vi "LateralControl.vi"(6 "output range":cluster{"output high":dbl, "output low":dbl}, 7 "PID Gains lateral":T1={"proportional gain (Kc)"=0.008, "integral time (Ti, min)"=0.0, "derivative time (Td, min)"=-0.07}, 9 "Waypoint 0":dbl[](array[numeric]), 10 "Waypoint 1":dbl[](array[numeric]), 11 "Position":dbl[](array[numeric])) -> (2 "y out":dbl, 3 "x out":dbl)   [LabVIEW 2018]
uses:
  <vilib>/Analysis/coordinate.llb/Wrap Angle (scalar).vi
  <vilib>/Analysis/coordinate.llb/2D Cartesian Coordinate Rotation (Scalar).vi
  <vilib>/Analysis/NI_AALPro.lvlib
  <vilib>/Analysis/NI_AAL_Angle.lvlib
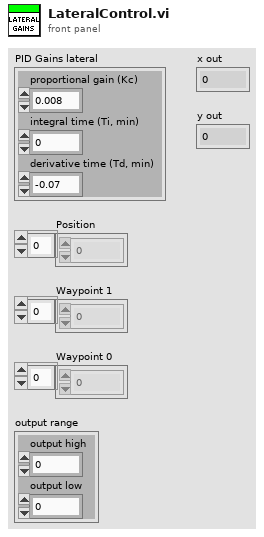
[diagram p1: front panel]
types:
  T1 = cluster{"proportional gain (Kc)":dbl, "integral time (Ti, min)":dbl, "derivative time (Td, min)":dbl}
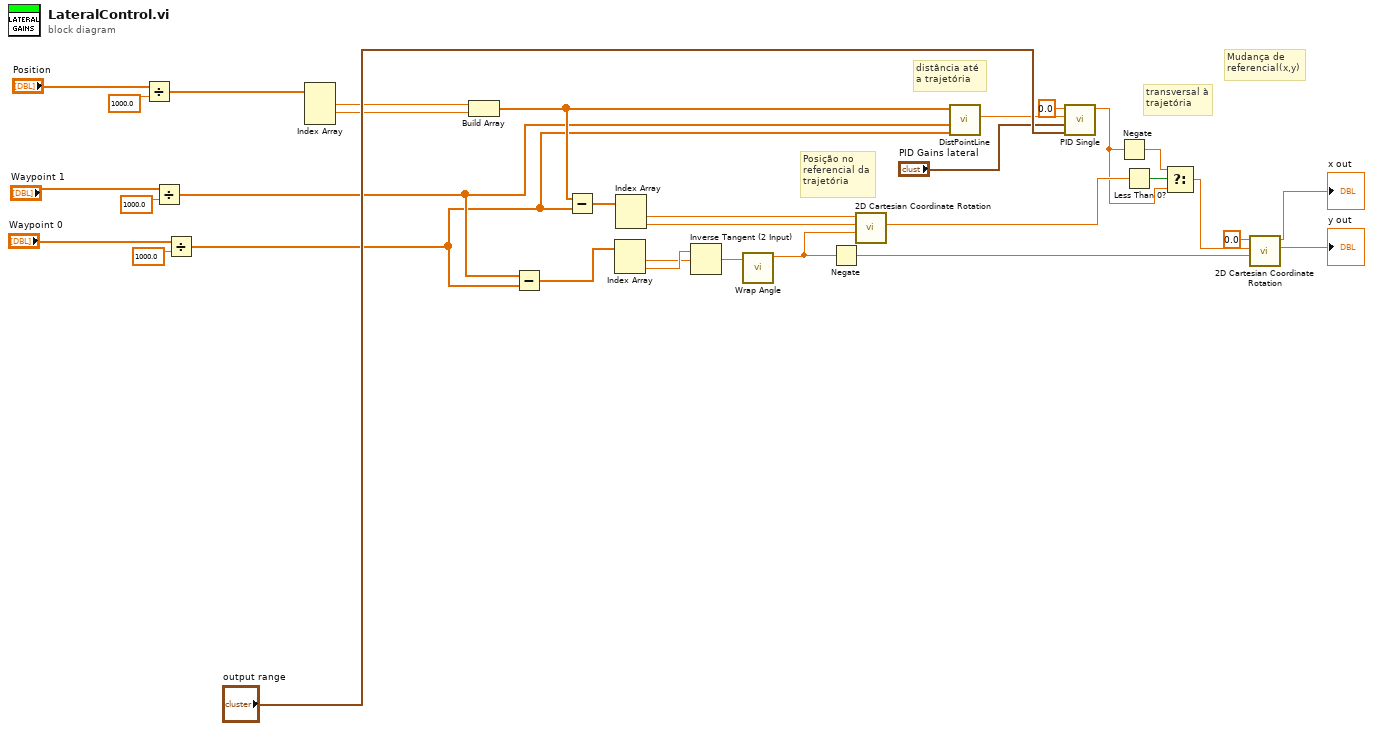
[diagram p0: block diagram]
diagram:
  # "Posição no \nreferencial da\ntrajetória"
  # "distância até \na trajetória"
  # "Mudança de \nreferencial(x,y)"
  # "transversal à\ntrajetória"
  n1 = Divide(x="Position", y=1000.0) -> (x/y=w9:dbl[])
  n2 = Divide(x="Waypoint 1", y=1000.0) -> (x/y=w5:dbl[])
  n3 = Divide(x="Waypoint 0", y=1000.0) -> (x/y=w1:dbl[])
  n4 = Index Array(array=w9) -> (element #1=w16:dbl, element #2=w17:dbl)  [unwired: 3 in, 1 out]
  n5 = Build Array(w16, w17) -> (w29:dbl[])
  n6 = Subtract(x=w5, y=w1) -> (x-y=w26:dbl[])
  n7 = Subtract(x=w29, y=w1) -> (x-y=w22:dbl[])
  n8 = Index Array(array=w26) -> (element #1=w14:dbl, element #2=w27:dbl)  [unwired: 2 in]
  n9 = Index Array(array=w22) -> (element #1=w23:dbl, element #2=w24:dbl)  [unwired: 2 in]
  n10 = Inverse Tangent (2 Input)(1:w14, 2:w27) -> (0:w15:dbl)
  n11 = call-poly <vilib>:"Wrap Angle.vi"("angle in"=w15) -> ("angle out"=w28:dbl)  [unwired: 9 in, 1 out]
  n12 = Negate(x=w28) -> (-x=w13:dbl)
  n13 = call-poly <vilib>:"2D Cartesian Coordinate Rotation.vi"("theta"=w28, "y"=w24, "x"=w23) -> ("y out"=w21:dbl)  [unwired: 6 in, 2 out]
  n14 = call "DistPointLine.vi"("P2"=w1, "P1"=w5, "Q"=w29) -> ("distance"=w10:dbl)  [unwired: 8 in]
  n15 = call "PID Single.vi"("Limits"="output range", "PID gains in"="PID Gains lateral", "Variable"=w10, "Setpoint"=0.0) -> ("Out"=w19:dbl)  [unwired: 7 in]
  n16 = Negate(x=w19) -> (-x=w18:dbl)
  n17 = Less Than 0?(x=w21) -> (x < 0?=w25:bool)
  n18 = Select(t=w18, s=w25, f=w19) -> (s? t:f=w20:dbl)
  n19 = call-poly <vilib>:"2D Cartesian Coordinate Rotation.vi"("theta"=w13, "y"=w20, "x"=0.0) -> ("y out"=→"y out":dbl, "x out"=→"x out":dbl)  [unwired: 6 in, 1 out]
